vi "Add Plugin Group Transfer Sections.vi"(8 "error in (no error)":errorcluster, 10 "framework configuration":T1, 11 "Item Ref in":T13 format="%.0x") -> (0 "error out":errorcluster, 3 "Item Ref out":T13 format="%.0x")   [LabVIEW 2017, in "DSF System Explorer.lvlib"]
uses:
  DSF System Explorer.lvlib
  <vilib>/NI Veristand/Custom Device API/Custom Device Item Ref.ctl
  DSF Core.lvlibp/Typedefs/DSF Engine Framework Configuration.ctl
  DSF Core.lvlibp/Typedefs/DSF Engine Plugin Configuration.ctl
  DSF Core.lvlibp/Typedefs/DSF Timing Info.ctl
  DSF Core.lvlibp/Typedefs/DSF Engine Plugin Thread Configuration.ctl
  DSF Core.lvlibp/Typedefs/DSF Settings Info.ctl
  DSF Core.lvlibp/Typedefs/DSF Engine Transfer Group Configuration.ctl
  DSF Core.lvlibp/Typedefs/DSF Direction.ctl
  DSF Core.lvlibp/Typedefs/DSF Engine Transfer Configuration.ctl
  DSF Core.lvlibp/Typedefs/DSF Byte Order.ctl
  DSF Core.lvlibp/Typedefs/DSF Engine Channel Configuration.ctl
  DSF Core.lvlibp/Typedefs/DSF Data Type.ctl
  DSF Core.lvlibp/Typedefs/DSF Timeout Behavior.ctl
  Shared/Plugin Page GUID.vi
  Shared/Group Page GUID.vi
  Shared/Transfer Page GUID.vi
  Shared/DSF Shared.lvlib
  <vilib>/NI Veristand/Custom Device API/Custom Device API.lvlib
  DSF Core.lvlibp
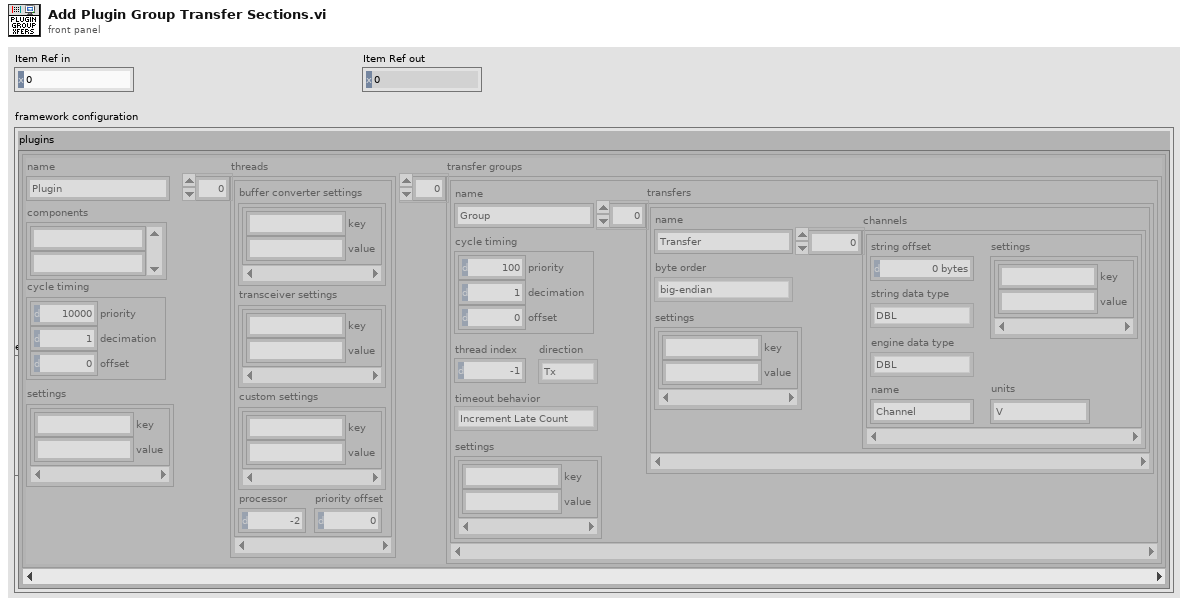
[diagram p1: front panel]
types:
  T1 = typedef "DSF Core.lvlibp/DSF Engine Framework Configuration.ctl" = cluster{"plugins":T2[]}
  T2 = typedef "DSF Core.lvlibp/DSF Engine Plugin Configuration.ctl" = cluster{"name":string, "components":string[], "cycle timing":T3, "threads":T4[], "transfer groups":T6[], "settings":T5}
  T3 = typedef "DSF Core.lvlibp/DSF Timing Info.ctl" = cluster{"priority":u64, "decimation":u64, "offset":u64}
  T4 = typedef "DSF Core.lvlibp/DSF Engine Plugin Thread Configuration.ctl" = cluster{"buffer converter settings":T5, "transceiver settings":T5, "custom settings":T5, "processor":i32, "priority offset":i16}
  T5 = typedef "DSF Core.lvlibp/DSF Settings Info.ctl" = cluster{"key":string, "value":string}[]
  T6 = typedef "DSF Core.lvlibp/DSF Engine Transfer Group Configuration.ctl" = cluster{"name":string, "direction":T7, "cycle timing":T3, "thread index":i32, "settings":T5, "transfers":T8[], "timeout behavior":T12}
  T7 = typedef "DSF Core.lvlibp/DSF Direction.ctl" = enum8{"Tx", "Rx"}
  T8 = typedef "DSF Core.lvlibp/DSF Engine Transfer Configuration.ctl" = cluster{"name":string, "byte order":T9, "settings":T5, "channels":T10[]}
  T9 = typedef "DSF Core.lvlibp/DSF Byte Order.ctl" = enum8{"big-endian", "little-endian"}
  T10 = typedef "DSF Core.lvlibp/DSF Engine Channel Configuration.ctl" = cluster{"string offset":u64, "string data type":T11, "engine data type":T11, "name":string, "settings":T5, "units":string}
  T11 = typedef "DSF Core.lvlibp/DSF Data Type.ctl" = enum8{"Bool", "SGL", "DBL", "I8", "I16", "I32", "I64", "U8", "U16", "U32", "U64"}
  T12 = typedef "DSF Core.lvlibp/DSF Timeout Behavior.ctl" = enum8{"Increment Late Count", "Throw Error"}
  T13 = typedef "Custom Device API.lvlib/Custom Device Item Ref.ctl" = u64
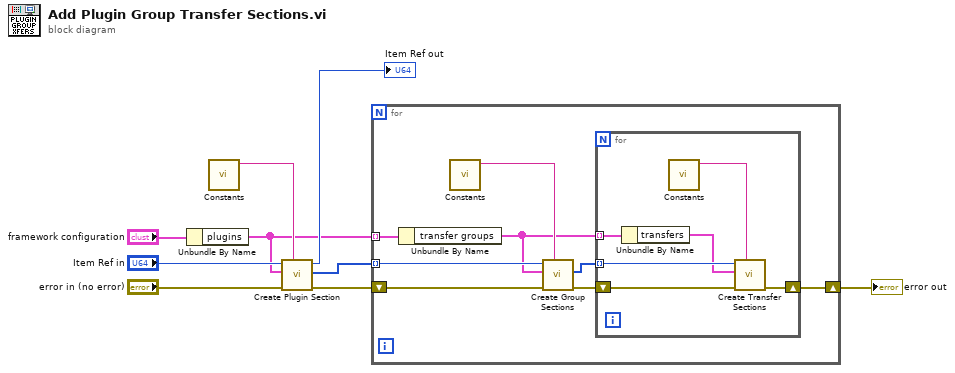
[diagram p0: block diagram]
diagram:
  n1 = Unbundle By Name("framework configuration") -> ("plugins"=w1:T2[])
  n2 = call-poly "Constants.vi"() -> ("Plugin GUID"=w2:string)  [unwired: 11 in]
  n3 = call "Create Plugin Section.vi"("GUID (Default Section)"=w2, "error in (no error)"="error in (no error)", "Plugins"=w1, "Item Ref in"="Item Ref in") -> ("error out"=w8:errorcluster, "Plugin Section refs"=w6:T13[], "Item Ref out"=→"Item Ref out":T13)  [unwired: 5 in]
  n4 = for {
    shift-right: [w15] -> w7
    shift-left: w8 -> [w12]
    tunnel: w6 -> [w17] mode=indexing
    tunnel: w1 -> [w13] mode=indexing
    n5 = Unbundle By Name(w13) -> ("transfer groups"=w10:T6[])
    n6 = call-poly "Constants.vi"() -> ("Group GUID"=w11:string)  [unwired: 11 in]
    n7 = call "Create Group Sections.vi"("GUID (Default Section)"=w11, "error in (no error)"=w12, "Transfer Groups"=w10, "Item Ref in"=w17) -> ("error out"=w16:errorcluster, "Group Section refs"=w14:T13[])  [unwired: 5 in, 1 out]
    n8 = for {
      shift-right: [w22] -> w15
      shift-left: w16 -> [w23]
      tunnel: w14 -> [w20] mode=indexing
      tunnel: w10 -> [w19] mode=indexing
      n9 = Unbundle By Name(w19) -> ("transfers"=w18:T8[])
      n10 = call-poly "Constants.vi"() -> ("Transfer GUID"=w21:string)  [unwired: 11 in]
      n11 = call "Create Transfer Sections.vi"("GUID (Default Section)"=w21, "error in (no error)"=w23, "Transfers"=w18, "Item Ref in"=w20) -> ("error out"=w22:errorcluster)  [unwired: 5 in, 2 out]
    }
  }
  "error out" <- w7
